vi "Actor Core.vi"(8 "error in":errorcluster, 11 "Nested in":refnum<class "Chat Window Interface.lvclass">) -> (0 "error out":errorcluster, 3 "Actor out":refnum<class "Actor.lvclass">)   [LabVIEW 2014, in "Chat Window Interface.lvlib" / "Chat Window Interface.lvclass"]
doc: "(<B>Filename</B>: Actor Framework.lvlib:Actor.lvclass:Actor Core.vi)\n\nReceives messages to the actor, reacts to them, and initiates any error handling that may shut the actor down.\n\nDescendant classes may override this VI to append parallel tasks for the actor to complete while it handles messages. Overrides use the Call Parent Method node."
uses:
  Chat Window Interface.lvclass
  <vilib>/ActorFramework/Actor/Actor.lvclass
  <vilib>/ActorFramework/Stop Msg/Stop Msg.lvclass
  Chat Window UI Controller/Chat Window UI Controller Messages/Send Status Updated Msg/Send Status Updated Msg.lvclass
  Chat Window UI Controller/Chat Window UI Controller Messages/Send Send Direct Message Msg/Send Send Direct Message Msg.lvclass
  Controls/Message Control.ctl
  Chat Window UI Controller/Chat Window UI Controller/Chat Window UI Controller.lvclass
panel:
  in  "My Status":string
  in  "Message":string
  in  "Send Message":bool
  in  "To":string(combo)
  out "Who's Online":string[](array[string])
  out "Messages":string
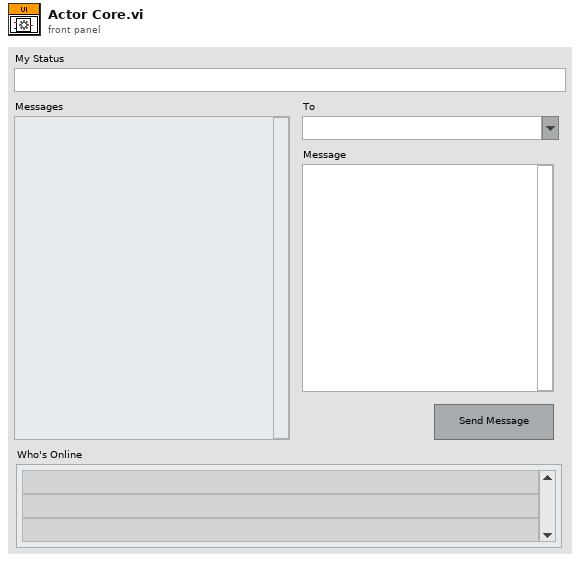
[diagram p1: front panel]
types:
  T1 = cluster{"Stop":refnum<user-event>, "Messages":refnum<user-event>, "OnlineStatus":refnum<user-event>}
  T2 = typedef "Message Control.ctl" = cluster{"From":string, "To":string, "Message":string}
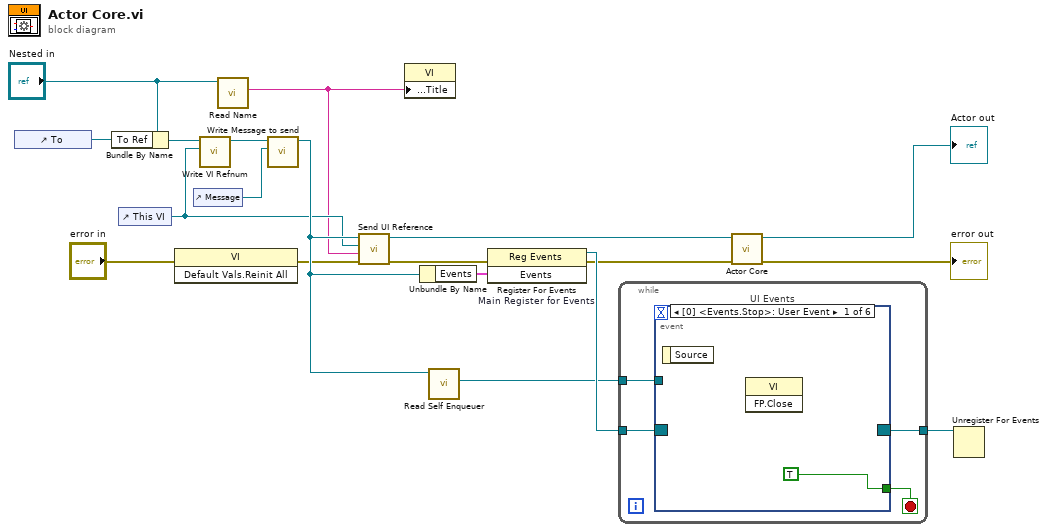
[diagram p0: block diagram]
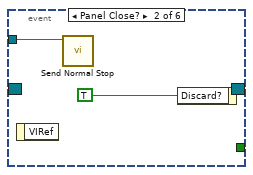
[diagram p2: hidden frame]
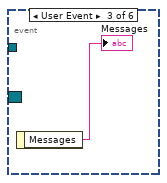
[diagram p3: hidden frame]
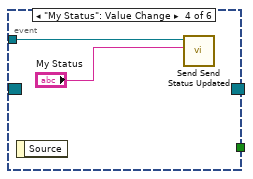
[diagram p4: hidden frame]
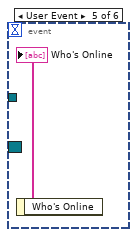
[diagram p5: hidden frame]
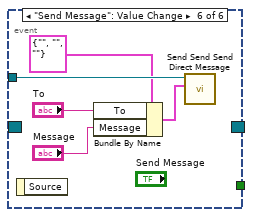
[diagram p6: hidden frame]
diagram:
  n1 = control-ref of="To"() -> (w11:refnum<vi>)
  n2 = Bundle By Name(cluster="Nested in", "To Ref"=w11) -> (w9:refnum<class "Chat Window Interface.lvclass">)
  n3 = control-ref of="This VI"() -> (w3:refnum<vi>)
  n4 = invoke class="VI" method="Default Vals.Reinit All"(error in="error in") -> (error out=w5:errorcluster)  [unwired: 2 in, 2 out]
  n5 = control-ref of="Message"() -> (w8:refnum<vi>)
  n6 = call "Write VI Refnum.vi"("VI Refnum"=w3, "Chat Window UI Controller in"=w9) -> ("Chat Window UI Controller out"=w7:refnum<class "Chat Window Interface.lvclass">)  [unwired: 8 in, 1 out]
  n7 = call "Read Name.vi"("Chat Window UI Controller in"="Nested in") -> ("Name"=w2:string)  [unwired: 8 in, 2 out]
  n8 = call "Write Message to send.vi"("Message to send"=w8, "Chat Window UI Controller in"=w7) -> ("Chat Window UI Controller out"=w6:refnum<class "Chat Window Interface.lvclass">)  [unwired: 8 in, 1 out]
  n9 = call "Send UI Reference.vi"("error in (no error)"=w5, "Name"=w2, "VI Refnum"=w3, "Chat Window UI Controller in"=w6) -> ("error out"=w4:errorcluster, "Chat Window UI Controller out"=w1:refnum<class "Chat Window Interface.lvclass">)  [unwired: 6 in]
  n10 = property class="VI"("Front Panel.Title"=w2) -> ()  [unwired: 2 in, 2 out]
  n11 = Unbundle By Name(w6) -> ("Events"=w16:T1)
  n12 = call <vilib>:"Read Self Enqueuer.vi"("Actor"=w6) -> ("Self Enqueuer"=w14:refnum<class "Message Enqueuer.lvclass">)  [unwired: 10 in]
  n13 = register-events "Main Register for Events"(error in=w4, w16) -> (reference out=w17:refnum<event-registration>, error out=w13:errorcluster)  [unwired: 1 in]
  n14 = while {
    tunnel: w17 -> [w23]
    tunnel: [w21] -> w15
    tunnel: w14 -> [w20]
    stop <- w22 stop-if-true
    n15 = event "UI Events" shown="[0] <Events.Stop>: User Event" {
      selector: w23 -> [_ _ _ _ _ _]
      dyn-events: [_ _ _ _ _ _] -> w21
      timeout: _ -> [_ _ _ _ _ _]
      tunnel: [TRUE _ _ _ _ _] -> w22
      tunnel: w20 -> [_ w25 _ w29 _ w35]
      event User Event {
        n16 = event-data() -> ()  [unwired: 1 in, 1 out]
        n17 = invoke class="VI" method="FP.Close"() -> ()  [unwired: 3 in, 3 out]
      }
      event Panel Close? {
        n18 = event-data() -> ()  [unwired: 1 in, 1 out]
        n19 = call <vilib>:"Send Normal Stop.vi"("Message Enqueuer"=w25) -> ()  [unwired: 10 in, 1 out]
        n20 = event-data("Discard?"=TRUE) -> ()  [unwired: 1 in, 1 out]
      }
      event User Event {
        n21 = event-data() -> ("Messages"=→"Messages":string)  [unwired: 1 in]
      }
      event "My Status": Value Change {
        n22 = event-data() -> ()  [unwired: 1 in, 1 out]
        n23 = call "Send Send Status Updated.vi"("Status"="My Status", "Message Enqueuer"=w29) -> ()  [unwired: 8 in, 2 out]
      }
      event User Event {
        n24 = event-data() -> ("Who's Online"=→"Who's Online":string[])  [unwired: 1 in]
      }
      event "Send Message": Value Change {
        n25 = event-data() -> ()  [unwired: 1 in, 1 out]
        n26 = Bundle By Name(cluster=T2 {"From"="", "To"="", "Message"=""} ("Message"), "To"="To", "Message"="Message") -> (w33:T2)
        n27 = call "Send Send Send Direct Message.vi"("Message"=w33, "Message Enqueuer"=w35) -> ()  [unwired: 8 in, 2 out]
      }
    }
  }
  n28 = call-parent "Actor Core.vi"("error in"=w13, "Actor in"=w1) -> ("error out"=→"error out":errorcluster, "Actor out"=→"Actor out":refnum<class "Actor.lvclass">)  [unwired: 8 in]
  n29 = Unregister For Events(event registration refnum=w15) -> ()  [unwired: 1 in, 1 out]
